vi "Remove_Spikes_sub.vi"(9 "Number of samples":i32, 10 "Time Trace in":dbl[](array[numeric]), 11 "Bkgnd Variance":dbl) -> (0 "Checked":bool, 2 "Time Trace out":dbl[](array[numeric]), 3 "Numeric out":i32)   [LabVIEW 2014]
uses:
  <vilib>/Analysis/NI_AALBase.lvlib
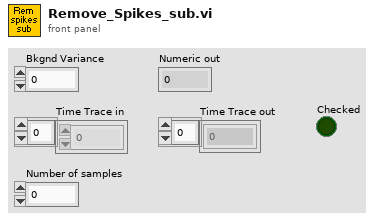
[diagram p1: front panel]
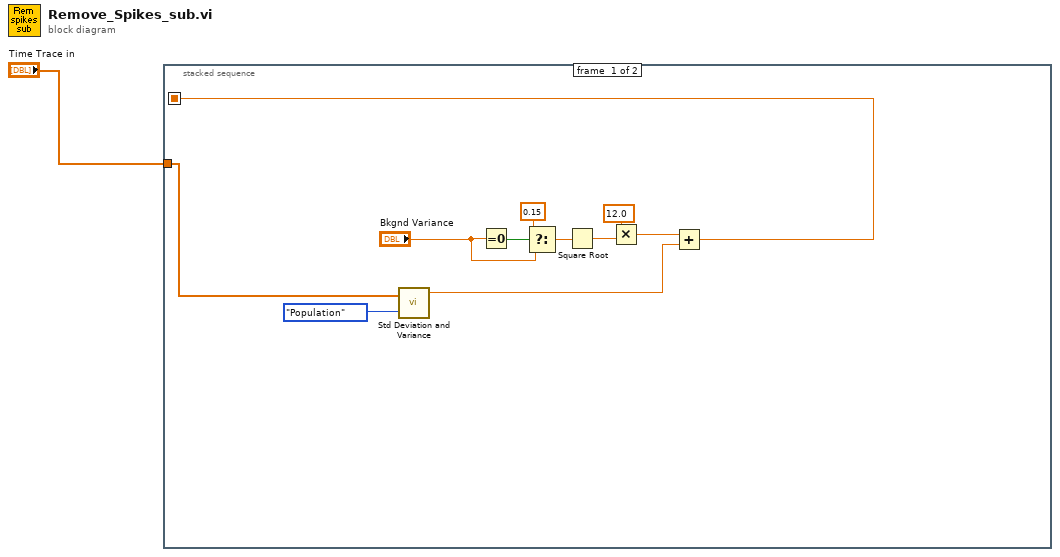
[diagram p0: block diagram]
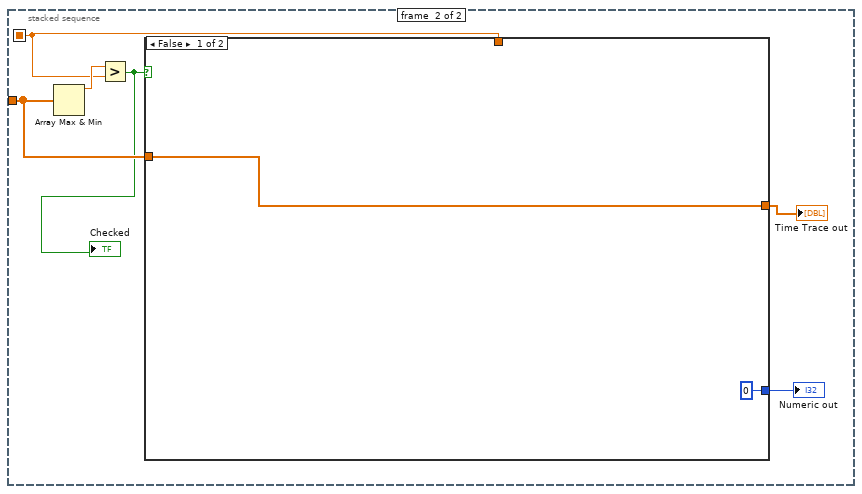
[diagram p2: hidden frame]
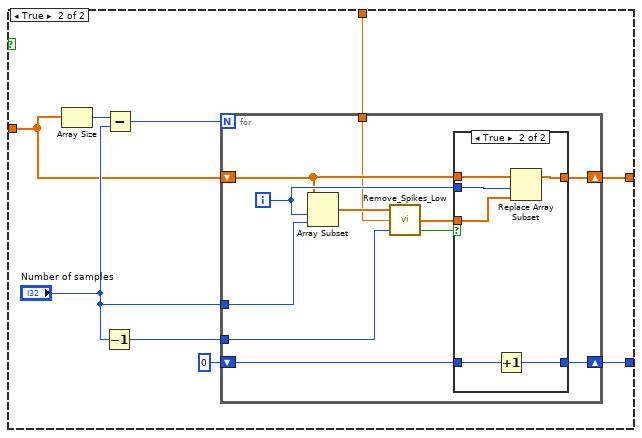
[diagram p3: hidden frame]
diagram:
  n1 = stacked-sequence {
    seq-local: [w3 _] -> [_ w14]
    tunnel: "Time Trace in" -> [w4 w15]
    frame #0 {
      n2 = call <vilib>:"Std Deviation and Variance.vi"("X"=w4, "Weighting (Sample)"=enum16{"Sample", "Population"}."Population") -> ("mean"=w7:dbl)  [unwired: 2 out]
      n3 = Equal To 0?(x="Bkgnd Variance") -> (x = 0?=w11:bool)
      n4 = Select(t=0.15, s=w11, f="Bkgnd Variance") -> (s? t:f=w9:dbl)
      n5 = Square Root(x=w9) -> (sqrt(x)=w6:dbl)
      n6 = Multiply(x=12.0 ("y"), y=w6) -> (x*y=w12:dbl)
      n7 = Add(x=w12, y=w7) -> (x+y=w3:dbl)
    }
    frame #1 {
      n8 = Array Max & Min(array=w15) -> (max value=w16:dbl)  [unwired: 3 out]
      n9 = Greater?(x=w16, y=w14) -> (0:w13:bool)
      "Checked" <- w13
      n10 = case shown="False" w13 {
        tunnel: [0 w27] -> w18
        tunnel: [w20 w26] -> w17
        tunnel: w14 -> [_ w22]
        tunnel: w15 -> [w20 w21]
        frame False {
        }
        frame True {
          n11 = Array Size(array=w21) -> (size(s)=w24:i32)
          n12 = Decrement(x="Number of samples") -> (x-1=w23:i32)
          n13 = Subtract(x=w24, y="Number of samples") -> (x-y=w25:i32)
          n14 = for {
            N: w25 -> [_]
            shift-right: [w33] -> w26
            shift-left: w21 -> [w34]
            tunnel: "Number of samples" -> [w40]
            tunnel: w23 -> [w39]
            tunnel: w22 -> [w32]
            shift-right: [w31] -> w27
            shift-left: 0 -> [w30]
            i -> [w36]
            n15 = Array Subset(array=w34, index=w36, length=w40) -> (w38:dbl[])
            n16 = call "Remove_Spikes_Low.vi"("index"=w39, "Background noise"=w32, "Time Trace"=w38) -> ("Spike"=w37:bool, "Filtered Time Trace"=w35:dbl[])  [unwired: 1 out]
            n17 = case shown="True" w37 {
              tunnel: w36 -> [_ w48]
              tunnel: w35 -> [_ w47]
              tunnel: w34 -> [w42 w46]
              tunnel: [w42 w45] -> w33
              tunnel: [w41 w43] -> w31
              tunnel: w30 -> [w41 w44]
              frame False {
              }
              frame True {
                n18 = Increment(x=w44) -> (x+1=w43:i32)
                n19 = Replace Array Subset(array=w46, new element=w47, index=w48) -> (w45:dbl[])
              }
            }
          }
        }
      }
      "Numeric out" <- w18
      "Time Trace out" <- w17
    }
  }
